vi "dio_driver.vi"(7 "Func":enum16{"Init", "Read", "Write", "Exit"}(ring), 8 "error in (no error)":errorcluster, 10 "Output":bool[](array[boolean])) -> (0 "error out":errorcluster, 2 "Inputs":bool[](array[boolean]), 3 "All Ok?":bool)   [LabVIEW 2014]
uses:
  <vilib>/Utility/error.llb/Error Cluster From Error Code.vi
  <vilib>/ErrorRing/Error Ring.xnode
  C:/Windows/System32/inpout32.dll
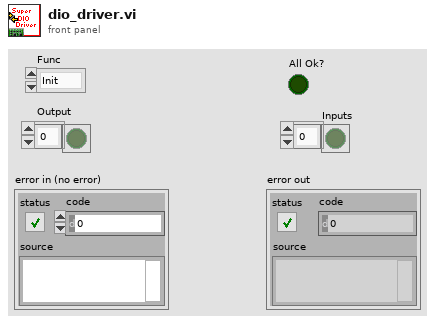
[diagram p1: front panel]
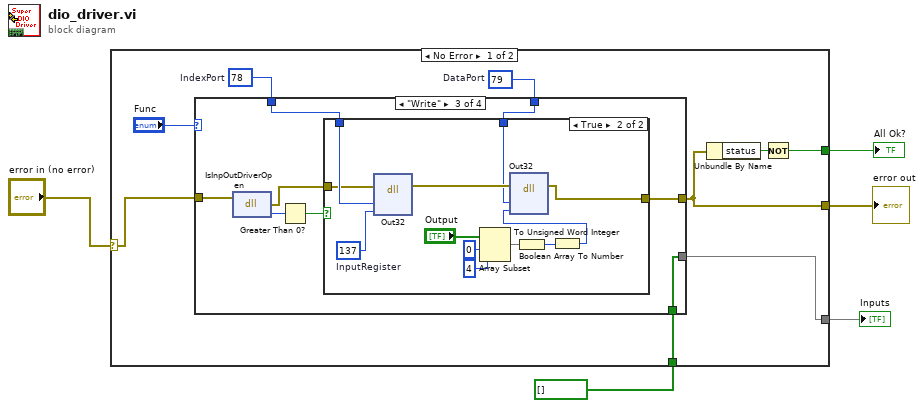
[diagram p0: block diagram]
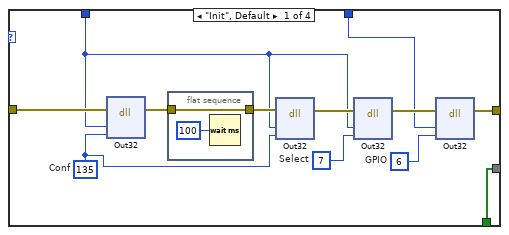
[diagram p2: hidden frame]
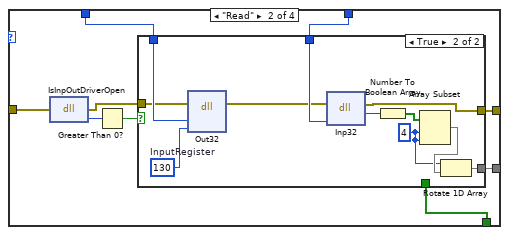
[diagram p3: hidden frame]
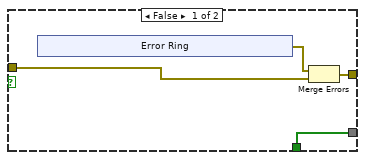
[diagram p4: hidden frame]
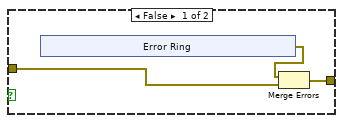
[diagram p5: hidden frame]
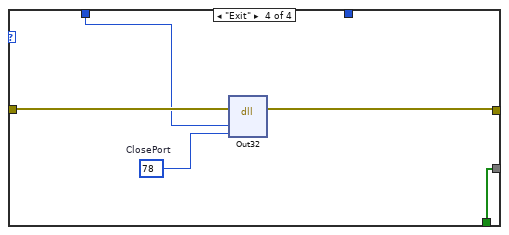
[diagram p6: hidden frame]
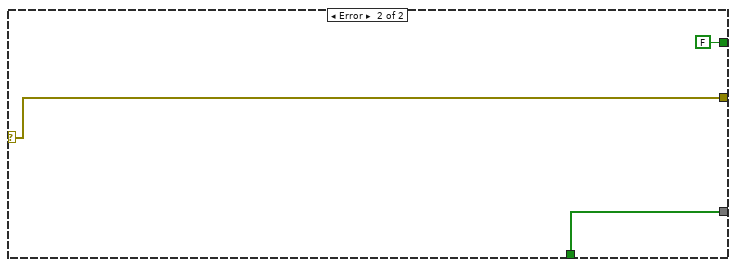
[diagram p7: hidden frame]
diagram:
  n1 = case shown="No Error" "error in (no error)" {
    selector: "error in (no error)" -> [w6 w91]
    tunnel: [w11 w91] -> w5
    tunnel: [w9 FALSE] -> w4
    tunnel: [w8 w93] -> w3
    tunnel: bool[] [] -> [w7 w93]
    frame No Error {
      w13 = u16 78  # IndexPort
      w12 = u16 79  # DataPort
      n2 = case shown="\"Write\"" "Func" {
        tunnel: w6 -> [w26 w35 w64 w89]
        tunnel: [w21 w30 w59 w88] -> w11
        tunnel: w13 -> [w17 w34 w61 w87]
        tunnel: w12 -> [w16 w32 w60 _]
        tunnel: [w15 w31 w58 w86] -> w8
        tunnel: w7 -> [w15 w29 w58 w86]
        frame "Init", Default {
          w18 = u16 6  # GPIO
          w19 = u16 7  # Select
          w20 = u16 135  # Conf
          n3 = dll-call lib="C:/Windows/System32/inpout32.dll" fn="Out32" label="inpout32.dll:\nOut32"(error in=w26, "port_ID"=w17, "DataVal_Index"=w20) -> (error out=w25:errorcluster)  [unwired: 5 in, 1 out]
          n4 = flat-sequence {
            tunnel: [w27] -> w24
            tunnel: w25 -> [w27]
            frame #0 {
              n5 = Wait (ms)(milliseconds to wait=u32 100) -> ()  [unwired: 1 out]
            }
          }
          n6 = dll-call lib="C:/Windows/System32/inpout32.dll" fn="Out32" label="inpout32.dll:\nOut32"(error in=w24, "port_ID"=w17, "DataVal_Index"=w20) -> (error out=w23:errorcluster)  [unwired: 5 in, 1 out]
          n7 = dll-call lib="C:/Windows/System32/inpout32.dll" fn="Out32" label="inpout32.dll:\nOut32"(error in=w23, "port_ID"=w17, "DataVal_Index"=w19) -> (error out=w22:errorcluster)  [unwired: 5 in, 1 out]
          n8 = dll-call lib="C:/Windows/System32/inpout32.dll" fn="Out32" label="inpout32.dll:\nOut32"(error in=w22, "port_ID"=w16, "DataVal_Index"=w18) -> (error out=w21:errorcluster)  [unwired: 5 in, 1 out]
        }
        frame "Read" {
          n9 = dll-call lib="C:/Windows/System32/inpout32.dll" fn="IsInpOutDriverOpen" label="inpout32.dll:\nIsInpOutDriverOpen"(error in=w35) -> (error out=w33:errorcluster, "return type"=w37:u8)  [unwired: 2 in, 1 out]
          n10 = Greater Than 0?(x=w37) -> (x > 0?=w36:bool)
          n11 = case shown="True" w36 {
            tunnel: w34 -> [_ w57]
            tunnel: w33 -> [w38 w56]
            tunnel: w32 -> [_ w55]
            tunnel: [w41 w48] -> w31
            tunnel: [w40 w47] -> w30
            tunnel: w29 -> [w41 _]
            frame False {
              n12 = xnode "Error Ring"() -> ("error out"=w39:errorcluster)
              n13 = Merge Errors(w39, w38) -> (w40:errorcluster)
            }
            frame True {
              w49 = 4 ("index")
              w53 = u16 130  # InputRegister
              n14 = dll-call lib="C:/Windows/System32/inpout32.dll" fn="Out32" label="inpout32.dll:\nOut32"(error in=w56, "port_ID"=w57, "DataVal_Index"=w53) -> (error out=w54:errorcluster)  [unwired: 5 in, 1 out]
              n15 = dll-call lib="C:/Windows/System32/inpout32.dll" fn="Inp32" label="inpout32.dll:\nInp32"(error in=w54, "port_ID"=w55) -> (error out=w47:errorcluster, "return read"=w52:u16)  [unwired: 3 in, 1 out]
              n16 = Number To Boolean Array(number=w52) -> (Boolean array=w51:bool[])
              n17 = Array Subset(array=w51, index=w49, length=w49) -> (w50:bool[])
              n18 = Rotate 1D Array(1:w50, 2:w49) -> (0:w48:bool[])
            }
          }
        }
        frame "Write" {
          n19 = dll-call lib="C:/Windows/System32/inpout32.dll" fn="IsInpOutDriverOpen" label="inpout32.dll:\nIsInpOutDriverOpen"(error in=w64) -> (error out=w62:errorcluster, "return type"=w65:u8)  [unwired: 2 in, 1 out]
          n20 = Greater Than 0?(x=w65) -> (x > 0?=w63:bool)
          n21 = case shown="True" w63 {
            tunnel: w61 -> [_ w85]
            tunnel: w62 -> [w66 w84]
            tunnel: w60 -> [_ w81]
            tunnel: [w68 w74] -> w59
            frame False {
              n22 = xnode "Error Ring"() -> ("error out"=w67:errorcluster)
              n23 = Merge Errors(w67, w66) -> (w68:errorcluster)
            }
            frame True {
              w83 = u16 137  # InputRegister
              n24 = dll-call lib="C:/Windows/System32/inpout32.dll" fn="Out32" label="inpout32.dll:\nOut32"(error in=w84, "port_ID"=w85, "DataVal_Index"=w83) -> (error out=w82:errorcluster)  [unwired: 5 in, 1 out]
              n25 = Array Subset(array="Output", index=0, length=4) -> (w80:bool[])
              n26 = Boolean Array To Number(Boolean array=w80) -> (number=w76:u32)
              n27 = To Unsigned Word Integer(number=w76) -> (unsigned 16bit integer=w75:u16)
              n28 = dll-call lib="C:/Windows/System32/inpout32.dll" fn="Out32" label="inpout32.dll:\nOut32"(error in=w82, "port_ID"=w81, "DataVal_Index"=w75) -> (error out=w74:errorcluster)  [unwired: 5 in, 1 out]
            }
          }
        }
        frame "Exit" {
          w90 = u16 78  # ClosePort
          n29 = dll-call lib="C:/Windows/System32/inpout32.dll" fn="Out32" label="inpout32.dll:\nOut32"(error in=w89, "port_ID"=w87, "DataVal_Index"=w90) -> (error out=w88:errorcluster)  [unwired: 5 in, 1 out]
        }
      }
      n30 = Unbundle By Name(w11) -> ("status"=w10:bool)
      n31 = Not(x=w10) -> (.not. x?=w9:bool)
    }
    frame Error {
    }
  }
  "error out" <- w5
  "All Ok?" <- w4
  "Inputs" <- w3
